vi "Example XYGraph Mouse Zoom.vi"() -> ()   [LabVIEW 2014]
uses:
  <vilib>/ptbypt/NI_PtbyPt.lvlib
  Graph Extensions.lvlib
panel:
  out "XY Graph":cluster{dbl[], dbl[]}[](graph)
  # "Instructions: Position the mouse over the graph, and use the scroll wheel to zoom in and out.  \n1. No modifiers, just straight scroll wheel.  This zooms on the X-Axis to zoom in and out\n2. SHIFT, changes the zoom to be on the Y-Axis\n3. CTRL, changes to a pan mode, sliding on the X-Axis with the scroll wheel\n4. CTRL SHIFT, pans on the Y-Axis with the scroll wheel"
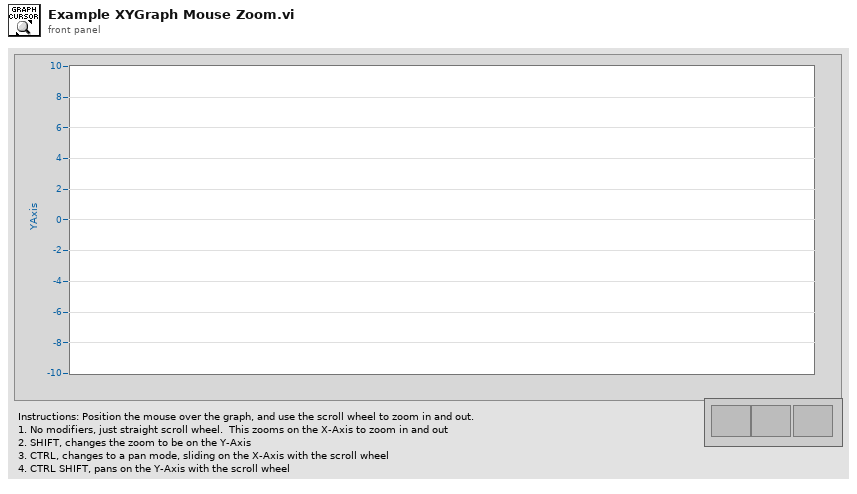
[diagram p1: front panel]
types:
  T1 = cluster{"Shift":bool, "Ctrl":bool, "Alt":bool, "Cmd":bool, "Opt":bool}
  T2 = typedef "LVPoint32TypeDef.ctl" = cluster{"Horizontal":i32, "Vertical":i32}
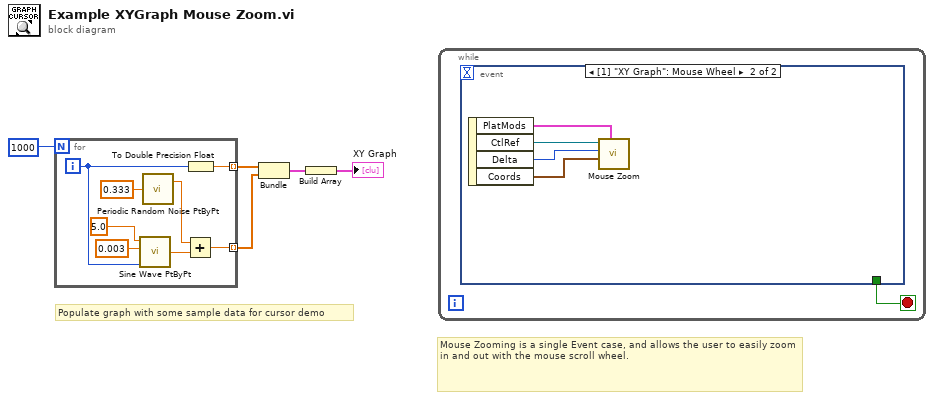
[diagram p0: block diagram]
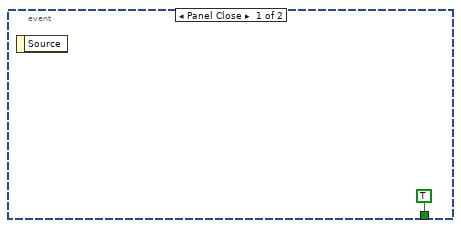
[diagram p2: hidden frame]
diagram:
  # "Populate graph with some sample data for cursor demo"
  # "Mouse Zooming is a single Event case, and allows the user to easily zoom in and out with the mouse scroll wheel."
  n1 = for {
    N: 1000 -> [_]
    tunnel: [w8] -> w4 mode=indexing
    tunnel: [w12] -> w5 mode=indexing
    i -> [w13]
    n2 = call <vilib>:"Sine Wave PtByPt.vi"("time"=w13, "frequency"=0.003, "amplitude"=5.0) -> ("sine wave"=w9:dbl)  [unwired: 1 in]
    n3 = call <vilib>:"Periodic Random Noise PtByPt.vi"("spectral amplitude"=0.333) -> ("periodic random noise"=w10:dbl)  [unwired: 3 in, 1 out]
    n4 = Add(x=w10, y=w9) -> (x+y=w8:dbl)
    n5 = To Double Precision Float(number=w13) -> (double precision float=w12:dbl)
  }
  n6 = Bundle(w5, w4) -> (w3:cluster{dbl[], dbl[]})  [unwired: 1 in]
  n7 = Build Array(w3) -> (→"XY Graph":cluster{dbl[], dbl[]}[])
  n8 = while {
    stop <- w14 stop-if-true
    n9 = event shown="[1] \"XY Graph\": Mouse Wheel" {
      selector: _ -> [_ _]
      dyn-events: _ -> [_ _]
      timeout: _ -> [_ _]
      tunnel: [TRUE _] -> w14
      event Panel Close {
        n10 = event-data() -> ()  [unwired: 1 in, 1 out]
      }
      event "XY Graph": Mouse Wheel {
        n11 = event-data() -> ("PlatMods"=w16:T1, "CtlRef"=w18:refnum<vi>, "Delta"=w19:i32, "Coords"=w17:T2)  [unwired: 1 in]
        n12 = call "Mouse Zoom.vi"("PlatMods"=w16, "XY"=w17, "Delta"=w19, "XY Graph"=w18) -> ()  [unwired: 8 in]
      }
    }
  }
